vi "Ctr Size Change.vi"(4 "CMC":refnum<vi>, 5 "배열 2":refnum<vi>[](array[refnum]), 6 "Proc":refnum<vi>, 7 "배열":refnum<vi>[](array[refnum]), 8 "error in (no error)":errorcluster caption="에러 입력(에러 없음)", 10 "탭 컨트롤":refnum<vi>, 11 "TabControl 입력":refnum<vi>) -> (0 "error out":errorcluster caption="에러 출력")   [LabVIEW 2020]
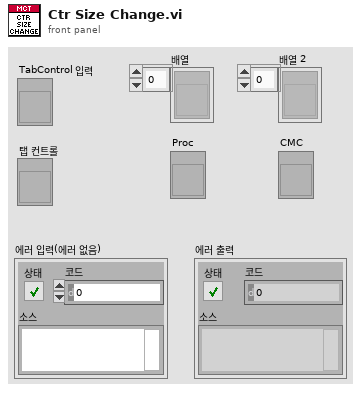
[diagram p1: front panel]
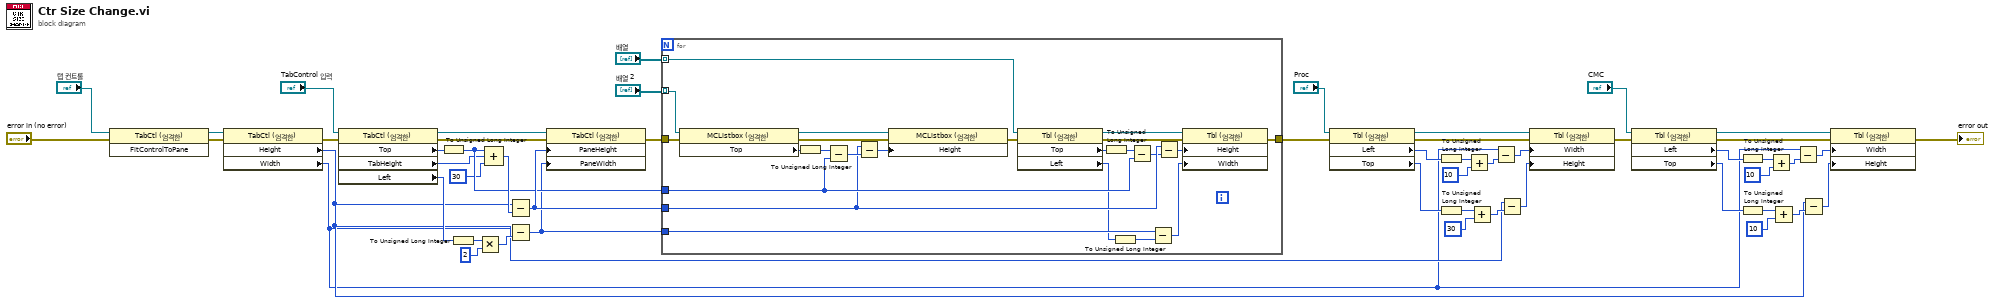
[diagram p0: block diagram]
diagram:
  n1 = invoke class="TabCtl (엄격한)" method="FitControlToPane"(reference="탭 컨트롤", error in="error in (no error)") -> (reference out=w52:refnum<vi>, error out=w51:errorcluster)  [unwired: 1 in, 1 out]
  n2 = property class="TabCtl (엄격한)"(reference=w52, error in=w51) -> (error out=w49:errorcluster, "Height"=w3:u32, "Width"=w2:u32)  [unwired: 1 out]
  n3 = property class="TabCtl (엄격한)"(reference="TabControl 입력", error in=w49) -> (reference out=w47:refnum<vi>, error out=w46:errorcluster, "Top"=w41:i32, "TabHeight"=w38:u32, "Left"=w36:i32)
  n4 = To Unsigned Long Integer(number=w41) -> (unsigned 32bit integer=w40:u32)
  n5 = To Unsigned Long Integer(number=w36) -> (unsigned 32bit integer=w35:u32)
  n6 = Multiply(x=w35, y=u32 2) -> (x*y=w34:u32)
  n7 = Compound Arithmetic op=ADD(w40, w38, u32 30 ("값")) -> (w48:u32)
  n8 = Subtract(x=w3, y=w48) -> (x-y=w42:u32)
  n9 = Subtract(x=w2, y=w34) -> (x-y=w32:u32)
  n10 = property class="TabCtl (엄격한)"(reference=w47, error in=w46, "PaneHeight"=w42, "PaneWidth"=w32) -> (error out=w43:errorcluster)  [unwired: 1 out]
  n11 = for {
    tunnel: "배열 2" -> [w74] mode=indexing
    tunnel: "배열" -> [w67] mode=indexing
    tunnel: w42 -> [w61]
    tunnel: w43 -> [w76]
    tunnel: w40 -> [w62]
    tunnel: [w58] -> w30
    tunnel: w32 -> [w56]
    n12 = property class="MCListbox (엄격한)"(reference=w74, error in=w76) -> (reference out=w73:refnum<vi>, error out=w75:errorcluster, "Top"=w71:i32)
    n13 = To Unsigned Long Integer(number=w71) -> (unsigned 32bit integer=w69:u32)
    n14 = Subtract(x=w69, y=w62) -> (x-y=w72:u32)
    n15 = Subtract(x=w61, y=w72) -> (x-y=w70:u32)
    n16 = property class="MCListbox (엄격한)"(reference=w73, error in=w75, "Height"=w70) -> (error out=w68:errorcluster)  [unwired: 1 out]
    n17 = property class="Tbl (엄격한)"(reference=w67, error in=w68) -> (reference out=w65:refnum<vi>, error out=w66:errorcluster, "Top"=w64:i32, "Left"=w55:i32)
    n18 = To Unsigned Long Integer(number=w64) -> (unsigned 32bit integer=w63:u32)
    n19 = To Unsigned Long Integer(number=w55) -> (unsigned 32bit integer=w54:u32)
    n20 = Subtract(x=w63, y=w62) -> (x-y=w60:u32)
    n21 = Subtract(x=w56, y=w54) -> (x-y=w57:u32)
    n22 = Subtract(x=w61, y=w60) -> (x-y=w59:u32)
    n23 = property class="Tbl (엄격한)"(reference=w65, error in=w66, "Height"=w59, "Width"=w57) -> (error out=w58:errorcluster)  [unwired: 1 out]
  }
  n24 = property class="Tbl (엄격한)"(reference="Proc", error in=w30) -> (reference out=w26:refnum<vi>, error out=w27:errorcluster, "Left"=w29:i32, "Top"=w28:i32)
  n25 = To Unsigned Long Integer(number=w29) -> (unsigned 32bit integer=w23:u32)
  n26 = To Unsigned Long Integer(number=w28) -> (unsigned 32bit integer=w21:u32)
  n27 = Add(x=w23, y=u32 10) -> (x+y=w22:u32)
  n28 = Add(x=w21, y=u32 30) -> (x+y=w19:u32)
  n29 = Subtract(x=w2, y=w22) -> (x-y=w24:u32)
  n30 = Subtract(x=w3, y=w19) -> (x-y=w25:u32)
  n31 = property class="Tbl (엄격한)"(reference=w26, error in=w27, "Width"=w24, "Height"=w25) -> (error out=w6:errorcluster)  [unwired: 1 out]
  n32 = property class="Tbl (엄격한)"(reference="CMC", error in=w6) -> (reference out=w1:refnum<vi>, error out=w9:errorcluster, "Left"=w7:i32, "Top"=w8:i32)
  n33 = To Unsigned Long Integer(number=w7) -> (unsigned 32bit integer=w12:u32)
  n34 = To Unsigned Long Integer(number=w8) -> (unsigned 32bit integer=w14:u32)
  n35 = Add(x=w12, y=u32 10) -> (x+y=w13:u32)
  n36 = Add(x=w14, y=u32 10) -> (x+y=w16:u32)
  n37 = Subtract(x=w2, y=w13) -> (x-y=w11:u32)
  n38 = Subtract(x=w3, y=w16) -> (x-y=w10:u32)
  n39 = property class="Tbl (엄격한)"(reference=w1, error in=w9, "Width"=w11, "Height"=w10) -> (error out=→"error out":errorcluster)  [unwired: 1 out]
